vi "V7310.Job.GetAll.vi"(6 "timeout ms (5000)":i32=5000, 8 "error in":errorcluster, 11 "Connection in":refnum<k5>) -> (0 "error out":errorcluster, 2 "Jobs":string[](array[string]), 3 "Connection out":refnum<k5>)   [LabVIEW 2016]
uses:
  LowLevel/V7310.Commands.ctl
  tools/Tma.lib/array.llb/Delete strings from array.vi
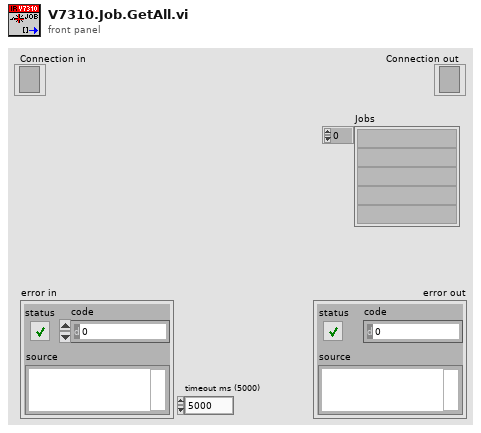
[diagram p1: front panel]
types:
  T1 = typedef "V7310.Commands.ctl" = enum16{"Start", "Stop", "GetStatus", "GetVarNames", "GetJobNames", "SetJob", "GetJob", "SetVars", "GetVars", "SetLayoutPosition", "SetRotation", "GetMessageID", "GetMessages", "ConfirmMessages", "DeleteMessages", "SetRTC", "GetRTC", "SetVarPosition", "SetIntensity", "GetIntensity", "SetStartTriggerDelay", "GetStartTriggerDelay", "SetStopTriggerDelay", "GetStopTriggerDelay", "SetConsecutiveTriggerDelay", "GetConsecutiveTriggerDelay", "SetMarkSpeed", "GetMarkSpeed"}
  T2 = typedef "V7310.ErrorLevels.ctl" = enum16{"OK", "Warning", "Error"}
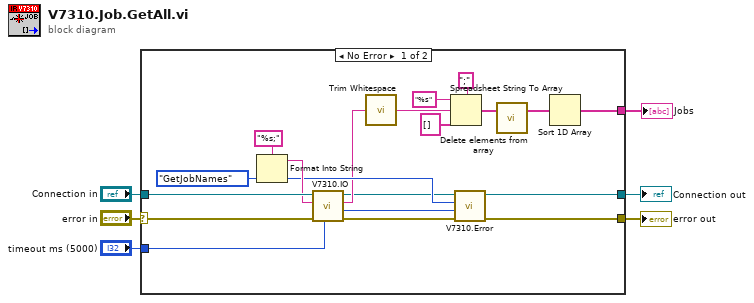
[diagram p0: block diagram]
diagram:
  n1 = case shown="No Error" "error in" {
    selector: "error in" -> [w23 w25]
    tunnel: "Connection in" -> [w24 w26]
    tunnel: [w11 w26] -> w5
    tunnel: "timeout ms (5000)" -> [w13 _]
    tunnel: [w12 w25] -> w2
    tunnel: [w10 _] -> w1
    frame No Error {
      w20 = V7310.Commands."GetJobNames" ("Cmd")
      n2 = Format Into String(format string="%s;", w20) -> (resulting string=w21:string)  [unwired: 2 in, 1 out]
      n3 = call "V7310.IO.vi"("timeout ms (5000)"=w13, "error in"=w23, "Data in"=w21, "Connection in"=w24) -> ("error out"=w18:errorcluster, "Error Level"=w19:T2, "Data out"=w14:string, "Connection out"=w11:refnum<k5>)  [unwired: 4 in]
      n4 = call <vilib>:"Trim Whitespace.vi"("string"=w14) -> ("trimmed string"=w9:string)  [unwired: 1 in]
      n5 = Spreadsheet String To Array(delimiter (Tab)=";", format string="%s", spreadsheet string=w9, array type (2D Dbl)=string[] [] ("StrArray")) -> (array=w8:string[])
      n6 = call "V7310.Error.vi"("error in"=w18, "Error Level"=w19, "Cmd"=w20) -> ("error out"=w12:errorcluster)  [unwired: 8 in]
      n7 = call-poly "Delete elements from array.vi"("strings in"=w8) -> ("strings out"=w7:string[])  [unwired: 2 in]
      n8 = Sort 1D Array(array=w7) -> (sorted array=w10:string[])
    }
    frame Error {
    }
  }
  "Connection out" <- w5
  "error out" <- w2
  "Jobs" <- w1
